vi "catalyst activation.vi"() -> ()   [LabVIEW 2014]
uses:
  <vilib>/ni845x/ni845x.llb/ni845xControl.ctl
  <vilib>/MakerHub/LINX/Public/Peripherals/Digital/Digital Write 1 Chan.vi
  <vilib>/MakerHub/LINX/Public/Peripherals/Analog/Analog Read N Chans.vi
  <vilib>/MakerHub/LINX/Public/Peripherals/Digital/Digital Write N Chans.vi
  <vilib>/MakerHub/LINX/Private/Local IO/LinxAnalogRead.vi
  <vilib>/MakerHub/LINX/Public/Utilities/Check Channel.vi
  <vilib>/MakerHub/LINX/Private/Local IO/LinxDigitalWrite.vi
  <vilib>/MakerHub/LINX/Private/Utilties/Generate Error.vi
  <vilib>/addons/control/pid/pid.llb/PID Control Input Filter (DBL).vi
  <vilib>/addons/control/pid/autopid.llb/PID Online Autotuning (Relay Feedback).vi
  <vilib>/addons/control/pid/NI_PID_autopid.lvlib
  <vilib>/addons/control/pid/NI_PID_pid.lvlib
  <vilib>/MakerHub/LINX/LMH-LINX.lvlib
panel:
  in  "Comprehensive Report File":string="C:\\Users\\Admin\\Documents\\Data\\catalyst_activation_suzuki_112816.xlsx"
  in  "Sample loop COMM":refnum<visa-resource-name>
  out "System Error":bool=TRUE
  out "Flowrate Sensor 4":dbl format="%#_13g"
  out "Flowrate Sensor 3":dbl format="%#_13g"
  out "Pressure 4":dbl format="%#_13g"
  out "Pressure 3":dbl format="%#_13g"
  out "Error Message":string
  out "Stop 2":bool=TRUE
  out "Pressure Chart":T1(graph)
  out "Flowrate Chart":T1(graph)
  in  "IR Sensor Device":T2
  in  "Arduino COMM Port":refnum<visa-resource-name>
  out "error out":errorcluster
  out "Temperature 7":dbl format="%#_g'C"
  out "Temperature 2":dbl format="%#_g'C"
  out "Temperature 6":dbl format="%#_g'C"
  out "Temperature 3":dbl format="%#_g'C"
  out "Temperature 1":dbl format="%#_g'C"
  out "Teperature Chart":T1(graph)
  out "Temperature 5":dbl format="%#_g'C"
  out "Temp SS? 4":bool=TRUE
  in  "Temperature Control 4":bool=TRUE
  in  "Temperature SP 4":dbl format="%#_g'C"
  out "Temperature 4":dbl format="%#_g'C"
  in  "SSR Duration 4":dbl
  out "Flowrate Sensor 2":dbl format="%#_13g"
  out "Flowrate Sensor 1":dbl format="%#_13g"
  out "Pressure 2":dbl format="%#_13g"
  out "Pressure 1":dbl format="%#_13g"
  in  "Stop":bool=TRUE
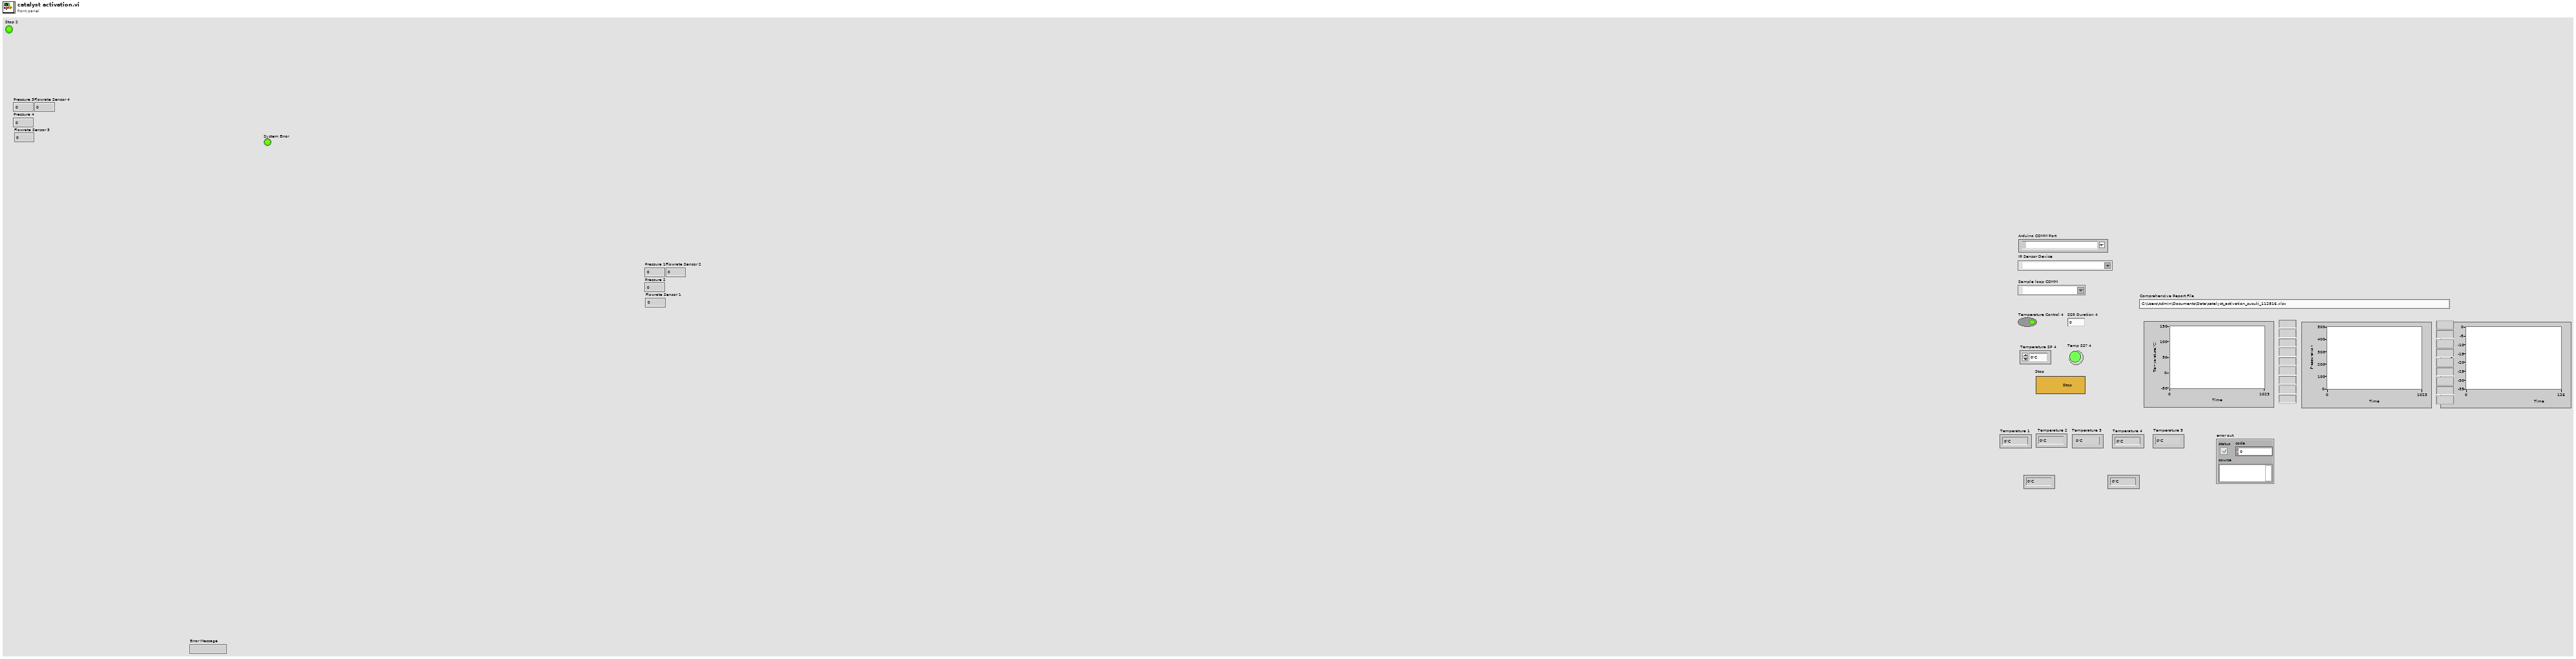
[diagram p1: front panel]
types:
  T1 = cluster{"[0]":dbl, "[1]":dbl, "[2]":dbl, "[3]":dbl, "[4]":dbl, "[5]":dbl, "[6]":dbl, "[7]":dbl, "[8]":dbl}
  T2 = typedef "ni845xControl.ctl" = refnum<k21>
  T3 = typedef "LMH-LINX.lvlib/LINX Ref.ctl" = cluster{"IO":T4, "Interface":T5, "LINX Device Config":T6}
  T4 = typedef "LMH-LINX.lvlib/Platform.ctl" = enum16{"Remote", "Local"}
  T5 = typedef "LMH-LINX.lvlib/Interface.ctl" = enum16{"Serial", "TCP"}
  T6 = typedef "LMH-LINX.lvlib/Device.lvlib/LINX Device Config.ctl" = cluster{"Interface":T5, "COM Port":refnum<visa-resource-name>, "TCP Configuration":T7, "Device Family":u8, "Device ID":u8, "Device Name":string, "TCP Ref":refnum<k5>, "Channels":T8}
  T7 = typedef "LMH-LINX.lvlib/Device.lvlib/TCP Config.ctl" = cluster{"IP Address":string, "Port":u16}
  T8 = typedef "LMH-LINX.lvlib/Channels.ctl" = cluster{"DI":u8[], "DO":u8[], "AI":u8[], "AO":u8[], "PWM":u8[], "QE":u8[], "UART":u8[], "I2C 2":u8[], "SPI":u8[], "CAN":u8[], "Servo":u8[], "AI Ref (V)":dbl, "AI Resolution (Bits)":u8, "AO Ref (V)":dbl, "AO Resolution (Bits)":u8}
  T9 = cluster{"Proportional gain Kc":dbl, "Integral time Ti (sec)":dbl, "Derivative time Ti (sec)":dbl}
  T10 = cluster{"type of controller":enum16{"P", "PI", "PID"}, "relay cycles":i32, "relay amplitude":dbl, "control specifications":enum16{"Fast", "Normal", "Slow"}, "PV noise level":dbl}
  T11 = cluster{"proportional gain (Kc)":dbl, "integral time (Ti, min)":dbl, "derivative time (Td, min)":dbl}
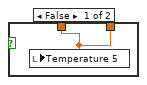
[diagram p4: hidden frame]
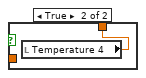
[diagram p5: hidden frame]
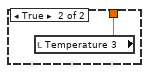
[diagram p6: hidden frame]
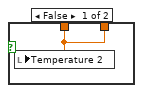
[diagram p7: hidden frame]
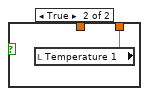
[diagram p8: hidden frame]
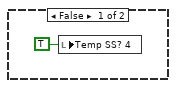
[diagram p9: hidden frame]
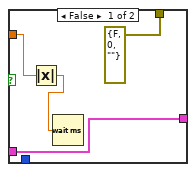
[diagram p10: hidden frame]
diagram:
  n1 = call <vilib>:"Initialize.vi"("Serial Port"="Arduino COMM Port") -> ("LINX Resource"=w2:T3)  [unwired: 8 in, 2 out]
  n2 = local read "IR Sensor Device"() -> (w4:T2)
  n3 = while {
    shift-right: [w28] -> _
    shift-left: w4 -> [w29]
    tunnel: errorcluster {"status"=FALSE, "code"=0, "source"=""} ("error out") -> [w27]
    stop <- w53 stop-if-true
    w44 = u8 7 items=["RAM IR raw  Ch1"=4, "RAM IR raw  Ch2"=5, "RAM T_A"=6, "RAM T_OBJ1"=7, "RAM T_OBJ2"=8, "EEPROM_To_max"=32, "EEPROM_To_min"=33, "EEPROM_PWM_CTRL"=34, "EEPROM_Ta_range"=35, "EEPROM_Emissivity_CorrCoeff"=36, "EEPROM_SMBus Address"=46, "EEPROM_ConfigReg"=37] ("Melexis_Cmmds")
    w46 = u8 7 items=["RAM IR raw  Ch1"=4, "RAM IR raw  Ch2"=5, "RAM T_A"=6, "RAM T_OBJ1"=7, "RAM T_OBJ2"=8, "EEPROM_To_max"=32, "EEPROM_To_min"=33, "EEPROM_PWM_CTRL"=34, "EEPROM_Ta_range"=35, "EEPROM_Emissivity_CorrCoeff"=36, "EEPROM_SMBus Address"=46, "EEPROM_ConfigReg"=37] ("Melexis_Cmmds")
    w45 = u8 7 items=["RAM IR raw  Ch1"=4, "RAM IR raw  Ch2"=5, "RAM T_A"=6, "RAM T_OBJ1"=7, "RAM T_OBJ2"=8, "EEPROM_To_max"=32, "EEPROM_To_min"=33, "EEPROM_PWM_CTRL"=34, "EEPROM_Ta_range"=35, "EEPROM_Emissivity_CorrCoeff"=36, "EEPROM_SMBus Address"=46, "EEPROM_ConfigReg"=37] ("Melexis_Cmmds")
    w50 = u8 7 items=["RAM IR raw  Ch1"=4, "RAM IR raw  Ch2"=5, "RAM T_A"=6, "RAM T_OBJ1"=7, "RAM T_OBJ2"=8, "EEPROM_To_max"=32, "EEPROM_To_min"=33, "EEPROM_PWM_CTRL"=34, "EEPROM_Ta_range"=35, "EEPROM_Emissivity_CorrCoeff"=36, "EEPROM_SMBus Address"=46, "EEPROM_ConfigReg"=37] ("Melexis_Cmmds")
    w55 = u8 7 items=["RAM IR raw  Ch1"=4, "RAM IR raw  Ch2"=5, "RAM T_A"=6, "RAM T_OBJ1"=7, "RAM T_OBJ2"=8, "EEPROM_To_max"=32, "EEPROM_To_min"=33, "EEPROM_PWM_CTRL"=34, "EEPROM_Ta_range"=35, "EEPROM_Emissivity_CorrCoeff"=36, "EEPROM_SMBus Address"=46, "EEPROM_ConfigReg"=37] ("Melexis_Cmmds")
    # "Bay 5 Temperature Read"
    # "Bay 4 Temperature Read"
    # "Bay 3 Temperature Read"
    # "Bay 2 Temperature Read"
    # "Bay 1 Temperature Read"
    n4 = local read "Stop"() -> (w53:bool)
    n5 = call "IRSensorNIRead.vi"("error in (no error)"=w27, "Melexis_Cmmds"=w55, "Address"=u8 1, "device reference"=w29) -> ("error out"=w26:errorcluster, "Temperature"=w56:dbl, "device reference out"=w52:T2)  [unwired: 5 in]
    n6 = Unbundle By Name(w26) -> ("status"=w25:bool)
    n7 = call-poly <vilib>:"PID Control Input Filter.vi"("input"=w56) -> ("output"=w24:dbl)  [unwired: 4 in]
    n8 = local write "error out"(w26) -> ()
    n9 = case shown="False" w25 {
      tunnel: w24 -> [w65 _]
      tunnel: [w65 w66] -> w23
      frame False {
        n10 = local write "Temperature 1"(w65) -> ()
      }
      frame True {
        n11 = local read "Temperature 1"() -> (w66:dbl)
      }
    }
    n12 = flat-sequence {
      tunnel: w52 -> [w75]
      tunnel: [w75] -> w51
      frame #0 {
        n13 = Wait (ms)(milliseconds to wait=u32 200) -> ()  [unwired: 1 out]
      }
    }
    n14 = call "IRSensorNIRead.vi"("error in (no error)"=w27, "Melexis_Cmmds"=w50, "Address"=u8 2, "device reference"=w51) -> ("error out"=w22:errorcluster, "Temperature"=w48:dbl, "device reference out"=w47:T2)  [unwired: 5 in]
    n15 = local write "error out"(w22) -> ()
    n16 = Unbundle By Name(w22) -> ("status"=w21:bool)
    n17 = call-poly <vilib>:"PID Control Input Filter.vi"("input"=w48) -> ("output"=w20:dbl)  [unwired: 4 in]
    n18 = case shown="True" w21 {
      tunnel: w20 -> [w63 _]
      tunnel: [w63 w64] -> w19
      frame False {
        n19 = local write "Temperature 2"(w63) -> ()
      }
      frame True {
        n20 = local read "Temperature 2"() -> (w64:dbl)
      }
    }
    n21 = flat-sequence {
      tunnel: w47 -> [w73]
      tunnel: [w73] -> w40
      frame #0 {
        n22 = Wait (ms)(milliseconds to wait=u32 200) -> ()  [unwired: 1 out]
      }
    }
    n23 = call "IRSensorNIRead.vi"("error in (no error)"=w27, "Melexis_Cmmds"=w45, "Address"=u8 3, "device reference"=w40) -> ("error out"=w15:errorcluster, "Temperature"=w35:dbl, "device reference out"=w39:T2)  [unwired: 5 in]
    n24 = local write "error out"(w15) -> ()
    n25 = Unbundle By Name(w15) -> ("status"=w16:bool)
    n26 = call-poly <vilib>:"PID Control Input Filter.vi"("input"=w35) -> ("output"=w18:dbl)  [unwired: 4 in]
    n27 = case shown="False" w16 {
      tunnel: w18 -> [w61 _]
      tunnel: [w61 w62] -> w17
      frame False {
        n28 = local write "Temperature 3"(w61) -> ()
      }
      frame True {
        n29 = local read "Temperature 3"() -> (w62:dbl)
      }
    }
    n30 = flat-sequence {
      tunnel: w39 -> [w71]
      tunnel: [w71] -> w37
      frame #0 {
        n31 = Wait (ms)(milliseconds to wait=u32 200) -> ()  [unwired: 1 out]
      }
    }
    n32 = call "IRSensorNIRead.vi"("error in (no error)"=w27, "Melexis_Cmmds"=w46, "Address"=u8 4, "device reference"=w37) -> ("error out"=w14:errorcluster, "Temperature"=w34:dbl, "device reference out"=w38:T2)  [unwired: 5 in]
    n33 = local write "error out"(w14) -> ()
    n34 = Unbundle By Name(w14) -> ("status"=w12:bool)
    n35 = flat-sequence {
      tunnel: w38 -> [w69]
      tunnel: [w69] -> w36
      frame #0 {
        n36 = Wait (ms)(milliseconds to wait=u32 200) -> ()  [unwired: 1 out]
      }
    }
    n37 = call-poly <vilib>:"PID Control Input Filter.vi"("input"=w34) -> ("output"=w13:dbl)  [unwired: 4 in]
    n38 = case shown="False" w12 {
      tunnel: w13 -> [w59 _]
      tunnel: [w59 w60] -> w11
      frame False {
        n39 = local write "Temperature 4"(w59) -> ()
      }
      frame True {
        n40 = local read "Temperature 4"() -> (w60:dbl)
      }
    }
    n41 = call "IRSensorNIRead.vi"("error in (no error)"=w27, "Melexis_Cmmds"=w44, "Address"=u8 5, "device reference"=w36) -> ("error out"=w10:errorcluster, "Temperature"=w33:dbl, "device reference out"=w32:T2)  [unwired: 5 in]
    n42 = flat-sequence {
      tunnel: w32 -> [w67]
      tunnel: [w67] -> w28
      frame #0 {
        n43 = Wait (ms)(milliseconds to wait=u32 200) -> ()  [unwired: 1 out]
      }
    }
    n44 = call-poly <vilib>:"PID Control Input Filter.vi"("input"=w33) -> ("output"=w8:dbl)  [unwired: 4 in]
    n45 = Unbundle By Name(w10) -> ("status"=w9:bool)
    n46 = case shown="True" w9 {
      tunnel: w8 -> [w57 _]
      tunnel: [w57 w58] -> w7
      frame False {
        n47 = local write "Temperature 5"(w57) -> ()
      }
      frame True {
        n48 = local read "Temperature 5"() -> (w58:dbl)
      }
    }
    n49 = local write "error out"(w10) -> ()
    n50 = Build Array(w23, w19, w17, w11, w7) -> (w31:dbl[])
    n51 = Array To Cluster(array=w31) -> (cluster=→"Teperature Chart":T1)
  }
  n52 = flat-sequence {
    tunnel: "Comprehensive Report File" -> [w77]
    frame #0 {
      n53 = script code="ExpNum = 0;\n\n%Setup output excel file\n% Opening Excel file and inputing first peaks headers if needed\ntry\n  xlApp = actxGetRunningServer('Excel.Application');\ncatch ME\n  xlApp = actxserver('Excel.Application');\nend\n\nxlApp.DisplayAlerts = false; \n\nxlWorkbook = xlApp.workbooks.Open(file, 0,false);\nxlApp.Visible = false;\nxlSheets = xlWorkbook.Sheets;\nxlSheetNamesArray = cell(xlSheets.Count, 1);\n\n\nfor i = 1:xlSheets.Count\n  xlSheetNamesArray{i} = xlSheets.Item(i).Name;\nend\n\n[~, idx1] = ismember('Time_Series_Conditions', xlSheetNamesArray);\nlastrow1 =2; lastcol1 = xlcolumnletter(6);"("file"=w77) -> ()  [unwired: 1 in, 1 out]
    }
    frame #1 {
      n54 = Multiply(x=60000.0, y=2.0) -> (x*y=w79:dbl)
      n55 = Wait (ms)(milliseconds to wait=w79) -> ()  [unwired: 1 out]
    }
    frame #2 {
      n56 = while {
        stop <- w81 stop-if-true
        n57 = Multiply(x=60000.0, y=1.0) -> (x*y=w82:dbl)
        n58 = Wait (ms)(milliseconds to wait=w82) -> ()  [unwired: 1 out]
        n59 = script code="temp_val1 = [ExpNum T3 Pres1 Pres2 F1 F2];\n\nlastrowStr = num2str(lastrow1);\nxlSheets.Item(idx1).Range(strcat('A',lastrowStr,':',lastcol1,lastrowStr)).Value2 = temp_val1;\nlastrow1 = lastrow1 + 1;"() -> ()  [unwired: 1 in, 1 out]
        n60 = local read "Stop"() -> (w81:bool)
      }
    }
  }
  n61 = while {
    tunnel: w2 -> [w87]
    stop <- w88 stop-if-true
    n62 = flat-sequence {
      tunnel: w87 -> [w94]
      tunnel: [w94] -> w86
      tunnel: w86 -> [w98]
      tunnel: [w98] -> w85
      tunnel: w85 -> [w99]
      frame #0 {
        n63 = Multiply(x=60000.0, y=8.0) -> (x*y=w91:dbl)
        n64 = Wait (ms)(milliseconds to wait=w91) -> ()  [unwired: 1 out]
      }
      frame #1 {
        n65 = call "NanoValve Load.vi"("VISA resource name"="Sample loop COMM") -> ()  [unwired: 10 in, 1 out]
      }
      frame #2 {
        n66 = Wait (ms)(milliseconds to wait=5000.0) -> ()  [unwired: 1 out]
      }
      frame #3 {
        n67 = call-poly <vilib>:"Digital Write.vi"("Output Value"=FALSE, "DO Channel"=u8 22, "LINX Resource"=w94) -> ()  [unwired: 7 in, 2 out]
      }
      frame #4 {
        n68 = Wait (ms)(milliseconds to wait=500.0) -> ()  [unwired: 1 out]
      }
      frame #5 {
        n69 = call-poly <vilib>:"Digital Write.vi"("Output Value"=TRUE, "DO Channel"=u8 22, "LINX Resource"=w99) -> ()  [unwired: 7 in, 2 out]
      }
      frame #6 {
        n70 = local read "Sample loop COMM"() -> (w102:refnum<visa-resource-name>)
        n71 = script code="ExpNum =  ExpNum +1;"() -> ()  [unwired: 1 in, 1 out]
        n72 = call "NanoValve Inject.vi"("VISA resource name"=w102) -> ()  [unwired: 10 in, 1 out]
      }
    }
    n73 = local read "Stop"() -> (w88:bool)
  }
  n74 = while {
    tunnel: w2 -> [w105]
    stop <- w104 stop-if-true
    n75 = Wait (ms)(milliseconds to wait=u32 300) -> ()  [unwired: 1 out]
    n76 = local read "Temperature Control 4"() -> (w103:bool)
    n77 = case shown="True" w103 {
      tunnel: w105 -> [_ w125]
      frame False {
        n78 = local write "Temp SS? 4"(TRUE ("Temp SS? 4")) -> ()
      }
      frame True {
        # "Bay 4 Temperature Controller"
        n79 = local read "Temperature SP 4"() -> (w108:dbl)
        n80 = local read "Temperature 4"() -> (w109:dbl)
        n81 = Subtract(x=w109, y=w108) -> (x-y=w111:dbl)
        n82 = Absolute Value(x=w111) -> (abs(x)=w113:dbl)
        n83 = Less Or Equal?(x=w113, y=1.2) -> (x <= y?=w110:bool)
        n84 = local write "Temp SS? 4"(w110) -> ()
        n85 = local read "SSR Duration 4"() -> (w114:dbl)
        n86 = call-poly <vilib>:"PID Online Autotuning.vi"("setpoint"=w108, "manipulated variable"=w114, "autotuning parameters"=T10 {"type of controller"=enum."PID", "relay cycles"=3, "relay amplitude"=1.0, "control specifications"=enum."Normal", "PV noise level"=0.1} ("Autotuning Parameters R1"), "process variable"=w109, "PID gains in"=T9 {"Proportional gain Kc"=0.38538, "Integral time Ti (sec)"=0.524375, "Derivative time Ti (sec)"=0.12585} ("PID gains 2")) -> ("setpoint out"=w116:dbl, "process variable out"=w117:dbl, "PID gains out"=w119:T11)  [unwired: 6 in, 2 out]
        n87 = call <vilib>:"PID Autotuning (Temperature).vi"("desired temperature"=w116, "measured temperature"=w117, "PID gains in"=w119, "output range"=cluster{"output high":dbl, "output low":dbl} {"output high"=3.0, "output low"=-1.0} ("Output range")) -> ("output"=w115:dbl)  [unwired: 12 in, 3 out]
        n88 = Multiply(x=1000.0, y=w115) -> (x*y=w123:dbl)
        n89 = Greater Than 0?(x=w123) -> (x > 0?=w124:bool)
        n90 = local write "SSR Duration 4"(w115) -> ()
        n91 = case shown="True" w124 {
          tunnel: [errorcluster {"status"=FALSE, "code"=0, "source"=""} ("error out") w134] -> _
          tunnel: 5 -> [_ w135]
          tunnel: [w128 w133] -> _
          tunnel: w125 -> [w128 w132]
          tunnel: w123 -> [w127 w131]
          frame False {
            n92 = Absolute Value(x=w127) -> (abs(x)=w129:dbl)
            n93 = Wait (ms)(milliseconds to wait=w129) -> ()  [unwired: 1 out]
          }
          frame True {
            n94 = call "TurnOnRelayArduino.vi"("channel"=w135, "duration"=w131, "LINX Resource"=w132) -> ("error out"=w134:errorcluster, "LINX Resource Out"=w133:T3)  [unwired: 7 in]
          }
        }
      }
    }
    n95 = local read "Stop"() -> (w104:bool)
  }
  n96 = while {
    tunnel: [w138] -> _
    tunnel: w2 -> [w138]
    tunnel: [w137] -> w3
    stop <- w187 stop-if-true
    w143 = 270
    w154 = 600
    w163 = 600
    # "Read Pressure and Flowrate"
    n97 = local read "Stop"() -> (w187:bool)
    n98 = call-poly <vilib>:"Analog Read.vi"("AI Channel(s)"=i32[] [12, 13, 14, 15], "LINX Resource"=w138) -> ("Voltages"=w185:dbl[], "LINX Resource"=w137:T3)  [unwired: 6 in, 2 out]
    n99 = Index Array(array=w185, index=3) -> (element=w177:dbl)
    n100 = Index Array(array=w185, index=2) -> (element=w178:dbl)
    n101 = Index Array(array=w185, index=1) -> (element=w179:dbl)
    n102 = Index Array(array=w185, index=0) -> (element=w180:dbl)
    n103 = call-poly <vilib>:"PID Control Input Filter.vi"("input"=w177) -> ("output"=w170:dbl)  [unwired: 4 in]
    n104 = call-poly <vilib>:"PID Control Input Filter.vi"("input"=w178) -> ("output"=w169:dbl)  [unwired: 4 in]
    n105 = call-poly <vilib>:"PID Control Input Filter.vi"("input"=w180) -> ("output"=w159:dbl)  [unwired: 4 in]
    n106 = call-poly <vilib>:"PID Control Input Filter.vi"("input"=w179) -> ("output"=w150:dbl)  [unwired: 4 in]
    n107 = Subtract(x=w159, y=0.065) -> (x-y=w160:dbl)
    n108 = Subtract(x=w150, y=0.065) -> (x-y=w151:dbl)
    n109 = Multiply(x=104.96 ("y"), y=w170) -> (x*y=w171:dbl)
    n110 = Multiply(x=104.96 ("y"), y=w169) -> (x*y=w174:dbl)
    n111 = Subtract(x=w171, y=24.077) -> (x-y=w141:dbl)
    n112 = Multiply(x=2, y=w163) -> (x*y=w165:i32)
    n113 = Divide(x=w165, y=3.3) -> (x/y=w161:dbl)
    n114 = Multiply(x=w160, y=w161) -> (x*y=w162:dbl)
    n115 = Subtract(x=w162, y=w163) -> (x-y=w145:dbl)
    n116 = Subtract(x=w174, y=24.077) -> (x-y=w142:dbl)
    n117 = Multiply(x=2, y=w154) -> (x*y=w156:i32)
    n118 = Divide(x=w156, y=3.3) -> (x/y=w152:dbl)
    n119 = Multiply(x=w151, y=w152) -> (x*y=w153:dbl)
    n120 = Subtract(x=w153, y=w154) -> (x-y=w144:dbl)
    n121 = Build Array(w145, w144) -> (w148:dbl[])
    n122 = Array To Cluster(array=w148) -> (cluster=→"Flowrate Chart":T1)
    n123 = Build Array(w142, w141) -> (w149:dbl[])
    n124 = local read "Temperature 3"() -> (w136:dbl)
    n125 = local write "Flowrate Sensor 3"(w145) -> ()
    n126 = local write "Flowrate Sensor 4"(w144) -> ()
    n127 = local write "Pressure 3"(w142) -> ()
    n128 = local write "Pressure 4"(w141) -> ()
    n129 = Array To Cluster(array=w149) -> (cluster=→"Pressure Chart":T1)
    n130 = Wait (ms)(milliseconds to wait=u32 500) -> ()  [unwired: 1 out]
    n131 = script code="MATLAB script"("F1"=w145, "F2"=w144, "Pres1"=w142, "Pres2"=w141, "T3"=w136) -> ()  [unwired: 1 in, 1 out]
    n132 = Greater?(x=w141, y=w143) -> (0:w139:bool)
    n133 = Greater?(x=w142, y=w143) -> (0:w140:bool)
    n134 = case shown="True" w140 {
      frame False {
      }
      frame True {
        w191 = TRUE ("Stop")
        n135 = local write "System Error"(w191) -> ()
        n136 = local write "Stop 2"(w191) -> ()
        n137 = local write "Error Message"("Pressure Sensor 1 readings above 250psi") -> ()
      }
    }
    n138 = case shown="True" w139 {
      frame False {
      }
      frame True {
        w189 = TRUE ("Stop")
        n139 = local write "System Error"(w189) -> ()
        n140 = local write "Stop 2"(w189) -> ()
        n141 = local write "Error Message"("Pressure Sensor 2 readings above 250psi") -> ()
      }
    }
  }
  n142 = call <vilib>:"Close.vi"("LINX Resource"=w3) -> ()  [unwired: 10 in, 1 out]
